vi "Climb Controller.vi"(8 "error in":errorcluster) -> ()   [LabVIEW 2019]
doc: "This VI executes continuously carrying out the current operation and responding to updates or new operations. It will often contain the timing or control code that is difficult to place directly in TeleOp. This VI generally opens all sensors and motors and isolates the rest of the robot code from knowing how the operations are carried out."
uses:
  Climb Operations.ctl
  Climb Setpoints.ctl
  <vilib>/Rock Robotics/Network Tables/NT Write Boolean.vi
  <vilib>/Rock Robotics/WPI/ThirdParty/REV Robotics/SPARK MAX/Typedef/Spark MAX Control Type.ctl
  <vilib>/Rock Robotics/WPI/Framework/Completion Status.ctl
panel:
  in  "Interactive Values":T1
  out "Current\nCmd":string
  in  "Buttons":cluster{"Execute Cmd":bool, "Abort Cmd":bool}
  out "Command Timing":cluster{"Start Time (ms)":u32, "Iterations":i32}
  out "Status":T3
  # "Tip: It may be helpful to observe inputs and sensor values.\nYou may also want to display tuning or debugging controls."
  # "Interactive Command: You may fill in the settings for a command\nand schedule it with the Execute button. You can observe and abort\nany command while fine tuning the code for the controller."
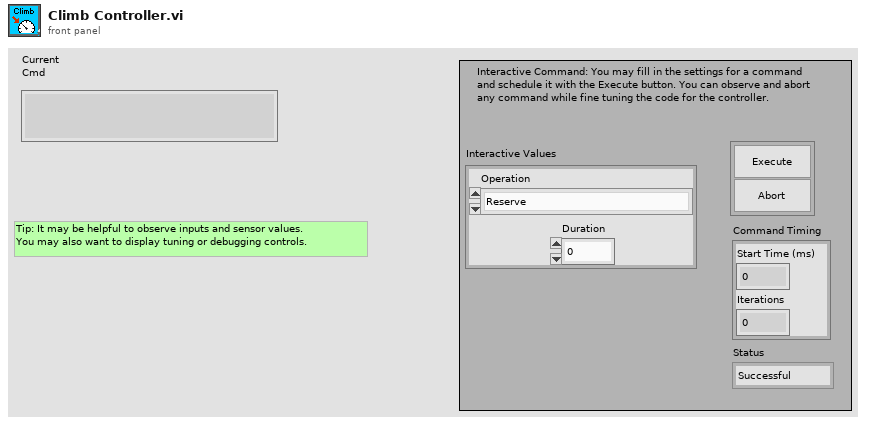
[diagram p1: front panel]
types:
  T1 = typedef "Climb Setpoints.ctl" = cluster{"Operation":T2, "Duration":dbl}
  T2 = typedef "Climb Operations.ctl" = enum16{"Reserve", "Read Current", "Immediate", "Go up", "Go down"}
  T3 = typedef "Completion Status.ctl" = enum16{"Successful", "Aborted", "Incomplete"}
  T4 = typedef "WPI_MotorControlDeviceRef.ctl" = cluster{"DeviceStatus":errorcluster, "Type":T5, "PWM":cluster{"PWM Channel":T6, "DeadBand":T7}, "CAN":cluster{"Device Number":u8, "SetOutput VI Ref":variant, "GetOutput VI Ref":variant, "Enable VI Ref":variant, "Disable VI Ref":variant, "Data":variant}, "Invert":bool, "DIO PWM":cluster{"PWM \"Enable\" Channel":T6, "DIOChannel":T8, "PWM Rate":dbl}}
  T5 = typedef "WPI_MotorControlType.ctl" = enum16{"PWM", "CAN", "DIO PWM"}
  T6 = typedef "FPGA_DIOPWMChannel.ctl" = enum8{"PWM 0", "PWM 1", "PWM 2", "PWM 3", "PWM 4", "PWM 5", "PWM 6", "PWM 7", "PWM 8", "PWM 9", "PWM MXP 0", "PWM MXP 1", "PWM MXP 2", "PWM MXP 3", "PWM MXP 4", "PWM MXP 5", "PWM MXP 6", "PWM MXP 7", "PWM MXP 8", "PWM MXP 9", "Invalid"}
  T7 = typedef "WPI_PWMDeadband.ctl" = cluster{"Name":string, "maxPositivePwm":i32, "minPositivePwm":i32, "centerPwm":i32, "maxNegativePwm":i32, "minNegativePwm":i32, "angularRange":u16}
  T8 = typedef "FPGA_DIOChannel.ctl" = enum8{"DIO 0", "DIO 1", "DIO 2", "DIO 3", "DIO 4", "DIO 5", "DIO 6", "DIO 7", "DIO 8", "DIO 9", "DIO MXP 0", "DIO MXP 1", "DIO MXP 2", "DIO MXP 3", "DIO MXP 4", "DIO MXP 5", "DIO MXP 6", "DIO MXP 7", "DIO MXP 8", "DIO MXP 9", "DIO MXP 10", "DIO MXP 11", "DIO MXP 12", "DIO MXP 13", "DIO MXP 14", "DIO MXP 15", "SPI Port CS1", "SPI Port CS2", "SPI Port CS3", "SPI Port MISO", "SPI Port MOSI", "Invalid"}
  T9 = typedef "Command Status Info.ctl" = cluster{"Name":string, "Status":T3, "notifier out":T10}
  T10 = typedef "Completion Notifier.ctl" = refnum<notifier>
  T11 = cluster{"Current Command":T1, "Command Timing":cluster{"Start Time (ms)":u32, "Iterations":i32}, "Command Arguments":cluster{"Command Info":T9, "Description":string, "Default Command":T1, "queue out":refnum<queue>, "Subsystem Name":string}}
  T12 = typedef "Spark MAX Control Type.ctl" = enum16{"Percent VBus", "Voltage", "Velocity", "Position", "Smart Motion", "Current", "Smart Velocity"}
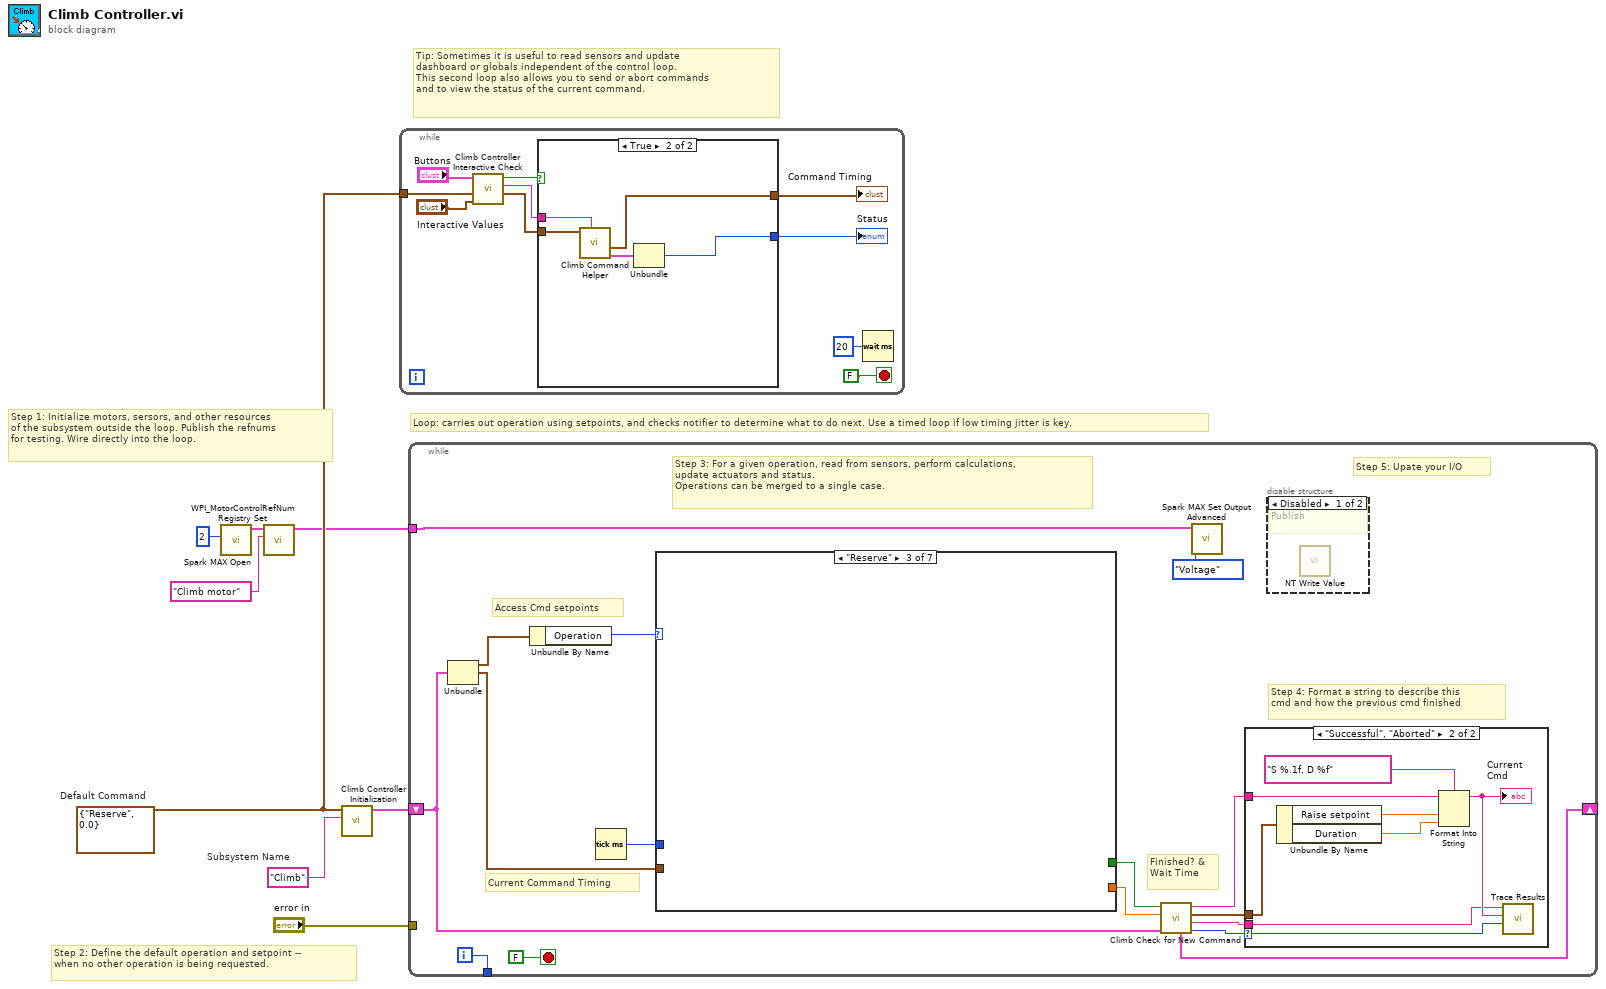
[diagram p0: block diagram]
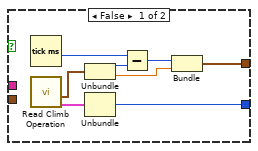
[diagram p2: hidden frame]
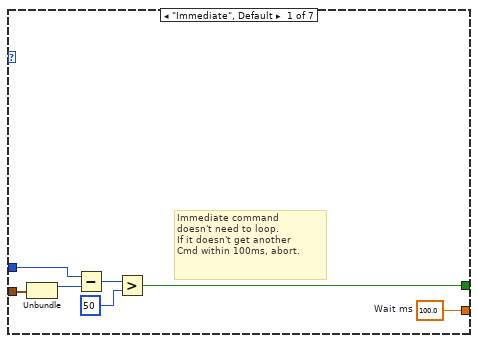
[diagram p5: hidden frame]
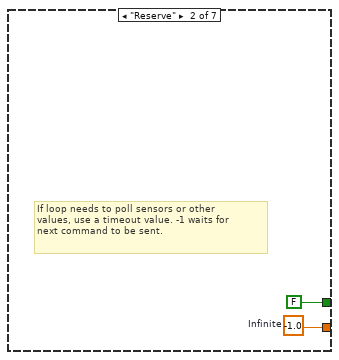
[diagram p6: hidden frame]
diagram:
  w5 = T1 {"Operation"=enum."Reserve", "Duration"=0.0}  # Default Command
  w6 = "Climb"  # Subsystem Name
  # "Tip: Sometimes it is useful to read sensors and update\ndashboard or globals independent of the control loop.\nThis second loop also allows you to send or abort commands\nand to view the status of the current command."
  # "Step 2: Define the default operation and setpoint --\nwhen no other operation is being requested."
  # "Step 1: Initialize motors, sersors, and other resources\nof the subsystem outside the loop. Publish the refnums\nfor testing. Wire directly into the loop."
  # "Loop: carries out operation using setpoints, and checks notifier to determine what to do next. Use a timed loop if low timing jitter is key."
  n1 = call <vilib>:"Spark MAX Open.vi"("Device Number"=u8 2) -> ("MotorControlDeviceRef"=w3:T4)  [unwired: 9 in, 1 out]
  n2 = call <vilib>:"WPI_MotorControlRefNum Registry Set.vi"("refnum name"="Climb motor", "MotorControlDevRef"=w3) -> ("MotorControlDevRef"=w1:T4)  [unwired: 8 in, 1 out]
  n3 = call "Climb Controller Initialization.vi"("Subsystem Name"=w6, "Default Command"=w5) -> ("Current Command"=w7:T11)  [unwired: 9 in]
  n4 = while {
    tunnel: w5 -> [w15]
    stop <- FALSE stop-if-true
    n5 = call "Climb Controller Interactive Check.vi"("Interactive Command in"="Interactive Values", "Default Command"=w15, "Buttons"="Buttons") -> ("Interactive Command out"=w12:T1, "Trace String"=w13:string, "Schedule"=w14:bool)  [unwired: 6 in]
    n6 = case shown="True" w14 {
      tunnel: [w26 w31] -> w11
      tunnel: w12 -> [_ w29]
      tunnel: [w22 w27] -> w10
      tunnel: w13 -> [_ w30]
      frame False {
        n7 = Tick Count (ms)() -> (millisecond timer value=w21:u32)
        n8 = call "Read Climb Operation.vi"() -> ("Command Info"=w19:T9, "SubSystem Data"=w20:T1)  [unwired: 9 in, 1 out]
        n9 = Unbundle(w20) -> ("Operation"=w25:T2, "Duration"=w23:dbl)
        n10 = Unbundle(w19) -> ("Status"=w26:T3)  [unwired: 2 out]
        n11 = Subtract(x=w21, y=w25) -> (x-y=w24:u32)
        n12 = Bundle(w24, "Duration"=w23) -> (w22:cluster{u32, "Duration":dbl})  [unwired: 1 in]
      }
      frame True {
        n13 = call "Climb Command Helper.vi"("Description"=w30, "SubSystem Data"=w29) -> ("Command Info Out"=w28:T9, "Command Timing"=w27:cluster{"Start Time (ms)":u32, "Iterations":i32})  [unwired: 7 in, 1 out]
        n14 = Unbundle(w28) -> ("Status"=w31:T3)  [unwired: 2 out]
      }
    }
    "Status" <- w11
    "Command Timing" <- w10
    n15 = Wait (ms)(milliseconds to wait=u32 20) -> ()  [unwired: 1 out]
  }
  n16 = while {
    shift-right: [w41] -> _
    shift-left: w7 -> [w34]
    tunnel: [w46] -> _
    tunnel: "error in" -> [_]
    tunnel: w1 -> [w32]
    i -> [w46]
    stop <- FALSE stop-if-true
    # "Step 5: Upate your I/O"
    # "Step 4: Format a string to describe this\ncmd and how the previous cmd finished"
    # "Current Command Timing"
    # "Access Cmd setpoints"
    # "Finished? &\nWait Time"
    # "Step 3: For a given operation, read from sensors, perform calculations,\nupdate actuators and status.\nOperations can be merged to a single case."
    n17 = Unbundle(w34) -> ("Current Command"=w45:T1, "Command Timing"=w42:cluster{"Start Time (ms)":u32, "Iterations":i32})  [unwired: 1 out]
    n18 = Unbundle By Name(w45) -> ("Operation"=w44:T2)
    n19 = Tick Count (ms)() -> (millisecond timer value=w43:u32)
    n20 = case shown="\"Climb Lower\"" w44 {
      tunnel: [w62 w64 _ _ _ _ _] -> w39
      tunnel: [w56 FALSE ("ignore previous (F)") _ _ _ _ _] -> w40
      tunnel: w42 -> [w58 _ _ _ _ _ _]
      tunnel: w43 -> [w57 _ _ _ _ _ _]
      frame "Immediate", Default {
        w62 = 100.0  # Wait ms
        # "Immediate command\ndoesn't need to loop.\nIf it doesn't get another\nCmd within 100ms, abort."
        n21 = Unbundle(w58) -> ("Start Time (ms)"=w61:u32)  [unwired: 1 out]
        n22 = Subtract(x=w57, y=w61) -> (x-y=w60:u32)
        n23 = Greater?(x=w60, y=u8 50 ("Left Motor")) -> (0:w56:bool)
      }
      frame "Reserve" {
        w64 = -1.0  # Infinite
        # "If loop needs to poll sensors or other\nvalues, use a timeout value. -1 waits for\nnext command to be sent."
      }
      frame "Reserve" {
      }
      frame "Read Current" {
      }
      frame "Read Current" {
      }
      frame "Go up" {
      }
      frame "Go down" {
      }
    }
    n24 = call "Climb Check for New Command.vi"("Current Command"=w34, "Wait time (ms)"=w39, "Finished?"=w40) -> ("Completion"=w35:T3, "Subsystem Name"=w36:string, "Current Command"=w37:T1, "Initial Trace String"=w38:string, "NextCommand"=w41:T11)  [unwired: 4 in]
    n25 = call <vilib>:"Spark MAX Set Output Advanced.vi"("Control Mode"=Spark_MAX_Control_Type."Voltage", "MotorControlDevRef"=w32) -> ()  [unwired: 8 in, 2 out]
    n26 = case shown="\"Successful\", \"Aborted\"" w35 {
      selector: w35 -> [_ w55]
      tunnel: w38 -> [_ w51]
      tunnel: w37 -> [_ w52]
      tunnel: w36 -> [_ w48]
      frame "Incomplete", Default {
        # "Continuing current command"
      }
      frame "Successful", "Aborted" {
        # "Report and setup for next command"
        n27 = Unbundle By Name(w52) -> ("Raise setpoint"=w54:dbl, "Duration"=w49:dbl)
        n28 = Format Into String(format string="S %.1f, D %f", initial string=w51, w54, w49) -> (resulting string=w50:string)  [unwired: 1 in, 1 out]
        "Current\nCmd" <- w50
        n29 = call <vilib>:"Trace Results.vi"("Status of previous command"=w55, "Description"=w50, "Subsystem"=w48) -> ()  [unwired: 9 in]
      }
    }
    n30 = disable-structure shown="Disabled" {
      frame Disabled {
        # "Publish"
        n31 = call-poly <vilib>:"NT Write Value.vi"() -> ()  [unwired: 11 in, 1 out]
      }
      frame Enabled {
      }
    }
  }
